vi "for_v0_v24.vi"() -> ()   [LabVIEW 2009]
panel:
  out "XY Graph":cluster{"Y":dbl[], "Y":dbl[]}[](graph)=[{"Y"=[0.0, 0.9659258262890683, 0.49999999999999994, -0.7071067811865475, -0.8660254037844386, 0.2588190451025211, 1.0, 0.2588190451025208, -0.8660254037844387, -0.7071067811865472, 0.5000000000000006, 0.9659258262890681, 6.123031769111886e-16, -0.9659258262890682, -0.5000000000000001, 0.7071067811865476, 0.8660254037844385, -0.25881904510252135, -1.0, -0.2588190451025197, 0.8660254037844394, 0.7071067811865464, -0.5000000000000016, -0.9659258262890678, -1.2246063538223773e-15, 0.965925826289068, 0.5000000000000007, -0.7071067811865471, -0.8660254037844388, 0.25881904510252074, 1.0, 0.2588190451025203, -0.866025403784439, -0.7071067811865468, 0.5000000000000011, 0.9659258262890679, -1.715804148066935e-15, -0.9659258262890688, -0.4999999999999981, 0.7071067811865492, 0.8660254037844373, -0.2588190451025236, -1.0, -0.25881904510251746, 0.8660254037844405, 0.7071067811865448, -0.5000000000000036, -0.9659258262890671, -2.4492127076447545e-15, 0.9659258262890678, 0.5000000000000017, -0.7071067811865464, -0.8660254037844394, 0.2588190451025196, 1.0, 0.25881904510252146, -0.8660254037844384, -0.7071067811865477, 0.5, 0.9659258262890682, -4.911977942445578e-16, -0.9659258262890684, -0.49999999999999917, 0.7071067811865483, 0.8660254037844379, -0.2588190451025224, -1.0, -0.25881904510251863, 0.8660254037844398, 0.7071067811865456, -0.5000000000000026, -0.9659258262890674, 3.43160829613387e-15, 0.9659258262890692, 0.4999999999999966, -0.7071067811865505, -0.8660254037844365, 0.25881904510252524, 1.0, 0.2588190451025158, -0.8660254037844414, -0.7071067811865436, 0.5000000000000051, 0.9659258262890666, -6.372018798023182e-15, -0.96592582628907, -0.49999999999999406, 0.7071067811865526, 0.8660254037844349, -0.2588190451025281, -1.0, -0.25881904510251297, 0.8660254037844428, 0.7071067811865415, -0.5000000000000077, -0.965925826289066, -4.898425415289509e-15, 0.9659258262890671, 0.5000000000000038, -0.7071067811865547, -0.8660254037844406, 0.25881904510253095, 1.0, 0.25881904510251014, -0.8660254037844372, -0.7071067811865394, 0.4999999999999979, 0.9659258262890652, 1.9580149134001967e-15, -0.9659258262890715, -0.5000000000000012, 0.7071067811865567, 0.8660254037844392, -0.2588190451025338, -1.0, -0.25881904510250725, 0.8660254037844386, 0.7071067811865372, -0.5000000000000004, -0.9659258262890644], "Y"=[1.0, 0.25881904510252074, -0.8660254037844387, -0.7071067811865477, 0.5000000000000001, 0.9659258262890682, 3.061515884555943e-16, -0.9659258262890683, -0.49999999999999983, 0.7071067811865478, 0.8660254037844383, -0.2588190451025216, -1.0, -0.25881904510252113, 0.8660254037844386, 0.7071067811865475, -0.5000000000000003, -0.9659258262890681, 8.579020740334675e-16, 0.9659258262890685, 0.49999999999999883, -0.7071067811865487, -0.8660254037844377, 0.2588190451025228, 1.0, 0.2588190451025217, -0.8660254037844383, -0.7071067811865479, 0.4999999999999998, 0.9659258262890683, -2.455988971222789e-16, -0.9659258262890684, -0.4999999999999994, 0.7071067811865482, 0.866025403784438, -0.2588190451025222, -1.0, -0.25881904510251885, 0.8660254037844397, 0.7071067811865458, -0.5000000000000023, -0.9659258262890675, 3.186009399011591e-15, 0.9659258262890692, 0.49999999999999684, -0.7071067811865503, -0.8660254037844366, 0.258819045102525, 1.0, 0.2588190451025229, -0.8660254037844377, -0.7071067811865487, 0.4999999999999987, 0.9659258262890686, 9.790074567000984e-16, -0.9659258262890681, -0.5000000000000004, 0.7071067811865474, 0.8660254037844386, -0.258819045102521, -1.0, -0.2588190451025201, 0.8660254037844392, 0.7071067811865467, -0.5000000000000012, -0.9659258262890679, 1.961403045189214e-15, 0.9659258262890689, 0.4999999999999979, -0.7071067811865495, -0.8660254037844372, 0.25881904510252385, 1.0, 0.2588190451025172, -0.8660254037844406, -0.7071067811865446, 0.5000000000000038, 0.9659258262890671, -4.901813547078526e-15, -0.9659258262890696, -0.49999999999999534, 0.7071067811865515, 0.8660254037844357, -0.2588190451025267, -1.0, -0.25881904510251436, 0.866025403784442, 0.7071067811865425, -0.5000000000000063, -0.9659258262890663, 7.842224048967839e-15, 0.9659258262890704, 0.4999999999999928, -0.7071067811865536, -0.8660254037844343, 0.2588190451025295, 1.0, 0.25881904510252524, -0.8660254037844365, -0.7071067811865405, 0.4999999999999966, 0.9659258262890655, 3.428220164344853e-15, -0.9659258262890711, -0.5000000000000026, 0.7071067811865557, 0.8660254037844398, -0.25881904510253234, -1.0, -0.2588190451025087, 0.8660254037844379, 0.7071067811865384, -0.49999999999999917, -0.9659258262890648, -4.878096624555406e-16, 0.9659258262890719, 0.5, -0.7071067811865578, -0.8660254037844384, 0.25881904510253523]}]
  in  "Nr de perioade cosinus":dbl(knob)=25.0 scale=0.0..25.0
  in  "stop":bool
  in  "Nr de perioade sinus":dbl(knob)=25.0 scale=0.0..25.0
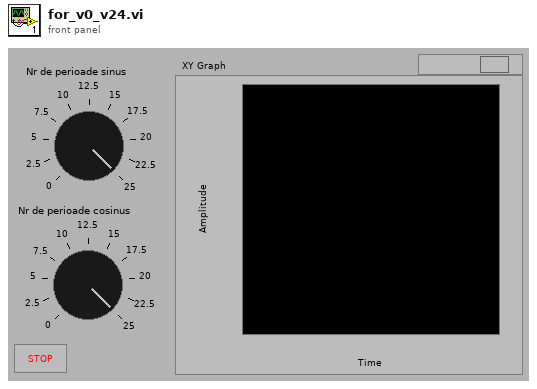
[diagram p1: front panel]
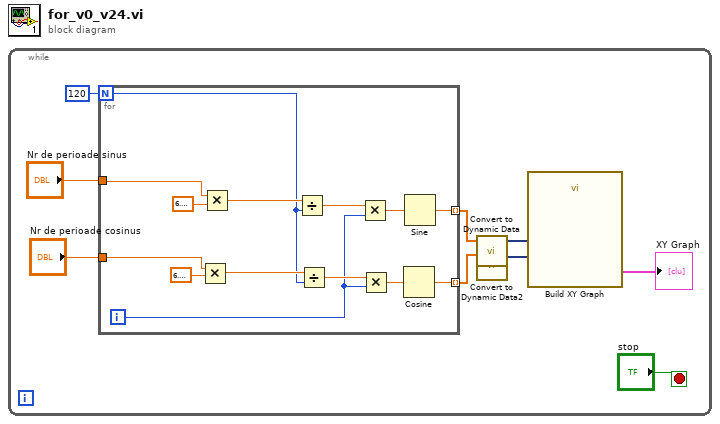
[diagram p0: block diagram]
diagram:
  n1 = while {
    stop <- "stop" stop-if-true
    n2 = for {
      N: 120 -> [w14]
      tunnel: [w23] -> w4 mode=indexing
      tunnel: "Nr de perioade sinus" -> [w19]
      tunnel: "Nr de perioade cosinus" -> [w16]
      tunnel: [w10] -> w2 mode=indexing
      i -> [w12]
      n3 = Multiply(x=w16, y=6.283185307179586) -> (x*y=w15:dbl)
      n4 = Multiply(x=w19, y=6.283185307179586) -> (x*y=w20:dbl)
      n5 = Divide(x=w20, y=w14) -> (x/y=w22:dbl)
      n6 = Divide(x=w15, y=w14) -> (x/y=w13:dbl)
      n7 = Multiply(x=w22, y=w12) -> (x*y=w21:dbl)
      n8 = Multiply(x=w13, y=w12) -> (x*y=w11:dbl)
      n9 = Cosine(x=w11) -> (cos(x)=w10:dbl)
      n10 = Sine(x=w21) -> (sin(x)=w23:dbl)
    }
    n11 = call "Convert to Dynamic Data"("Array"=w4) -> ("Dynamic Data Type"=w3:dynamicdata)  [unwired: 3 in]
    n12 = call "Convert to Dynamic Data2"("Array"=w2) -> ("Dynamic Data Type"=w1:dynamicdata)  [unwired: 3 in]
    n13 = call "Build XY Graph"("Y Input"=w1, "X Input"=w3) -> ("XY Graph"=→"XY Graph":cluster{"Y":dbl[], "Y":dbl[]}[])  [unwired: 8 in, 1 out]
  }
